vi "Select RT System.vi"(4 "Error In (no error)":errorcluster, 6 "Timeout ms (4000)":i32=4000, 7 "Display Mode":u16(ring) items=["All", "Configured only", "Unconfigured only"]) -> (0 "error out":errorcluster, 2 "MAC Address Out":string, 3 "IP Addresst Out":string)   [LabVIEW 2015]
panel:
  out "Slide":i32(slide) scale=0.0..100.0
  out "String":string="Please wait up to 30 Sec for system to search for remote RT targets."
  in  "Remote RT Systems":i32(listbox)
  in  "Cancel":bool
  in  "OK":bool
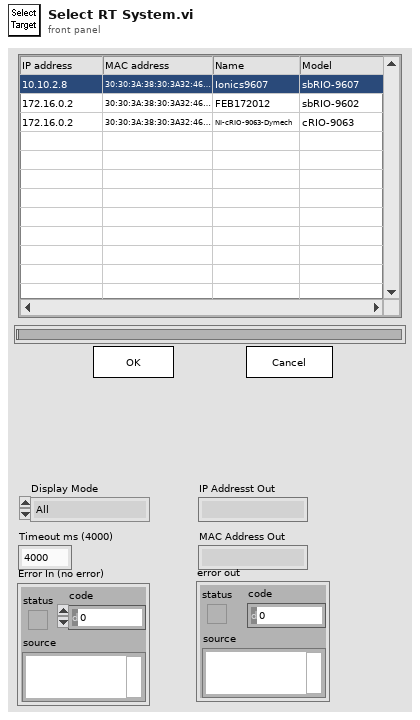
[diagram p1: front panel]
types:
  T1 = cluster{"IP Address":string, "MAC Address":string, "Hostname":string, "Model":string}[]
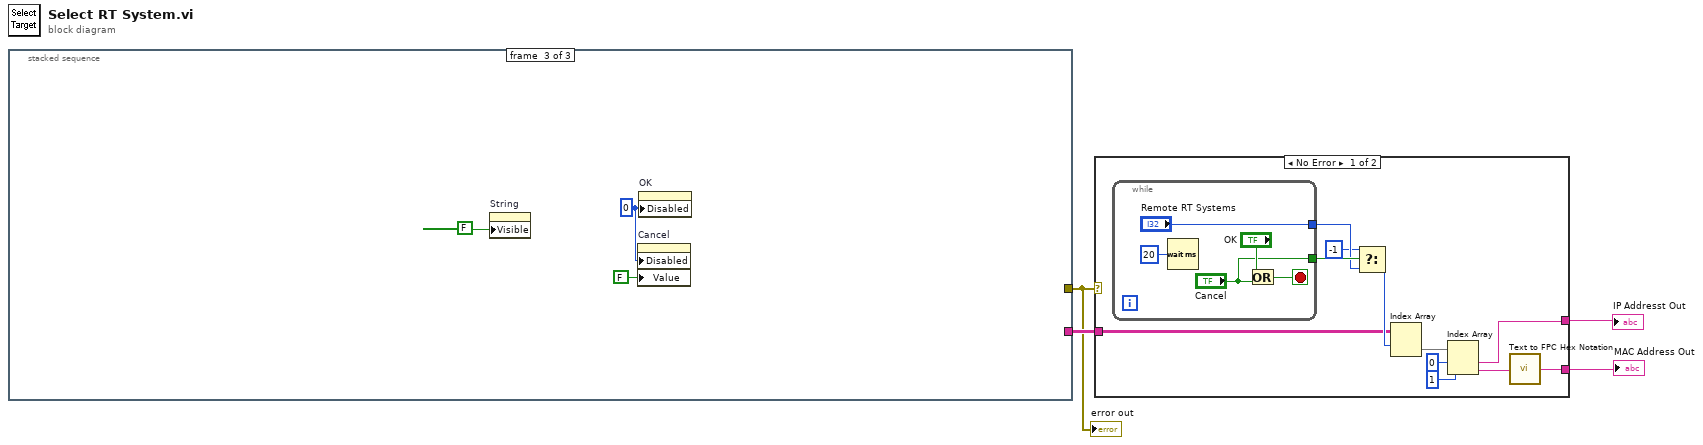
[diagram p0: block diagram]
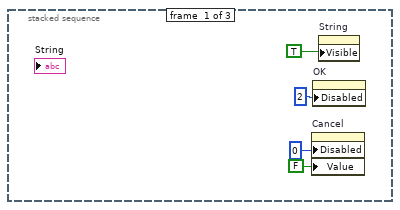
[diagram p2: hidden frame]
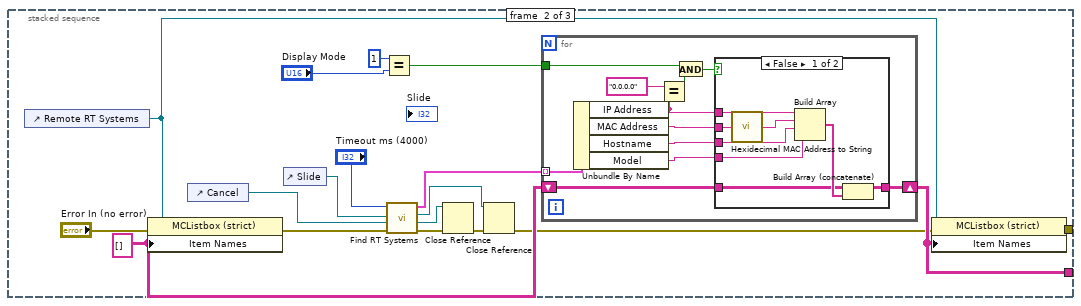
[diagram p3: hidden frame]
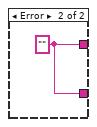
[diagram p5: hidden frame]
diagram:
  n1 = stacked-sequence {
    tunnel: [_ w25 _] -> w4
    tunnel: [_ w24 _] -> w3
    frame #0 {
      n2 = property on="Cancel" class="Bool (strict)"("Disabled"=u8 0, "Value"=FALSE ("Cancel")) -> ()  [unwired: 2 in, 2 out]
      n3 = property on="OK" class="Bool"("Disabled"=u8 2) -> ()  [unwired: 2 in, 2 out]
      n4 = property on="String" class="Str"("Visible"=TRUE) -> ()  [unwired: 2 in, 2 out]
    }
    frame #1 {
      w18 = string[][] []
      n5 = control-ref of="Remote RT Systems"() -> (w14:refnum<vi>)
      n6 = property class="MCListbox (strict)"(reference=w14, error in="Error In (no error)", "Item Names"=w18) -> (error out=w20:errorcluster)  [unwired: 1 out]
      n7 = control-ref of="Cancel"() -> (w13:refnum<vi>)
      n8 = control-ref of="Slide"() -> (w15:refnum<vi>)
      n9 = Equal?(x=u16 1, y="Display Mode") -> (x = y?=w21:bool)
      n10 = call "Find RT Systems.vi"("error in (no error)"=w20, "Cancel In Reference"=w13, "Progress Reference In"=w15, "Timeout ms (4000)"="Timeout ms (4000)") -> ("error out"=w26:errorcluster, "Progress Reference Out"=w9:refnum<vi>, "Cancel Out"=w10:refnum<vi>, "All RT Info"=w17:T1)  [unwired: 4 in]
      n11 = Close Reference(reference=w9, error in (no error)=w26) -> (error out=w11:errorcluster)
      n12 = Close Reference(reference=w10, error in (no error)=w11) -> (error out=w12:errorcluster)
      n13 = for {
        tunnel: w17 -> [w37] mode=indexing
        tunnel: w21 -> [w31]
        shift-right: [w28] -> w25
        shift-left: w18 -> [w27]
        n14 = Unbundle By Name(w37) -> ("IP Address"=w33:string, "MAC Address"=w34:string, "Hostname"=w36:string, "Model"=w35:string)
        n15 = Equal?(x="0.0.0.0", y=w33) -> (x = y?=w30:bool)
        n16 = And(x=w31, y=w30) -> (x .and. y?=w29:bool)
        n17 = case shown="False" w29 {
          tunnel: w33 -> [w45 _]
          tunnel: w36 -> [w44 _]
          tunnel: w35 -> [w43 _]
          tunnel: w34 -> [w42 _]
          tunnel: [w39 w46] -> w28
          tunnel: w27 -> [w38 w46]
          frame False {
            n18 = call <userlib>:"Hexidecimal MAC Address to String.vi"("MAC Address"=w42) -> ("MAC Address ("=w41:string)
            n19 = Build Array(w45, w41, w44, w43) -> (w40:string[])
            n20 = Build Array (concatenate)(w38, w40) -> (w39:string[][])
          }
          frame True {
          }
        }
      }
      n21 = property class="MCListbox (strict)"(reference=w14, error in=w12, "Item Names"=w25) -> (error out=w24:errorcluster)  [unwired: 1 out]
    }
    frame #2 {
      w49 = u8 0 ("Disabled")
      n22 = property on="String" class="Str"("Visible"=FALSE) -> ()  [unwired: 2 in, 2 out]
      n23 = property on="Cancel" class="Bool (strict)"("Disabled"=w49, "Value"=FALSE ("Cancel")) -> ()  [unwired: 2 in, 2 out]
      n24 = property on="OK" class="Bool"("Disabled"=w49) -> ()  [unwired: 2 in, 2 out]
    }
  }
  "error out" <- w3
  n25 = case shown="No Error" w3 {
    tunnel: w4 -> [w59 _]
    tunnel: [w52 w66] -> w2
    tunnel: [w50 w66] -> w1
    frame No Error {
      n26 = while {
        tunnel: ["Remote RT Systems"] -> w57
        tunnel: ["Cancel"] -> w58
        stop <- w64 stop-if-true
        n27 = Wait (ms)(milliseconds to wait=u32 20) -> ()  [unwired: 1 out]
        n28 = Or(x="OK", y="Cancel") -> (x .or. y?=w64:bool)
      }
      n29 = Select(t=-1, s=w58, f=w57) -> (s? t:f=w60:i32)
      n30 = Index Array(array=w59, index (row)=w60) -> (element=w55:string[])  [unwired: 1 in]
      n31 = Index Array(array=w55, index #1=0 ("index"), index #2=1 ("index")) -> (element #1=w52:string, element #2=w51:string)
      n32 = call <userlib>:"Text to FPC Hex Notation.vi"("Text string"=w51) -> ("Hex notation string"=w50:string)  [unwired: 14 out]
    }
    frame Error {
      w66 = ""
    }
  }
  "MAC Address Out" <- w1
  "IP Addresst Out" <- w2
